vi "Get.vi"(8 "error in (no error)":errorcluster, 9 "Parameter":string, 10 "Request":string, 11 "ByteGSWebAPI-V0 in":refnum<class "ByteGSWebAPI-V0.lvclass">) -> (0 "error out":errorcluster, 3 "ByteGSWebAPI-V0 out":refnum<class "ByteGSWebAPI-V0.lvclass">, 4 "body":string, 6 "headers":string)   [LabVIEW 2019, in "ByteGSWebAPI.lvlib" / "ByteGSWebAPI-V0.lvclass"]
uses:
  ByteGSWebAPI-V0.lvclass
  <vilib>/httpClient/LabVIEWHTTPClient.lvlib
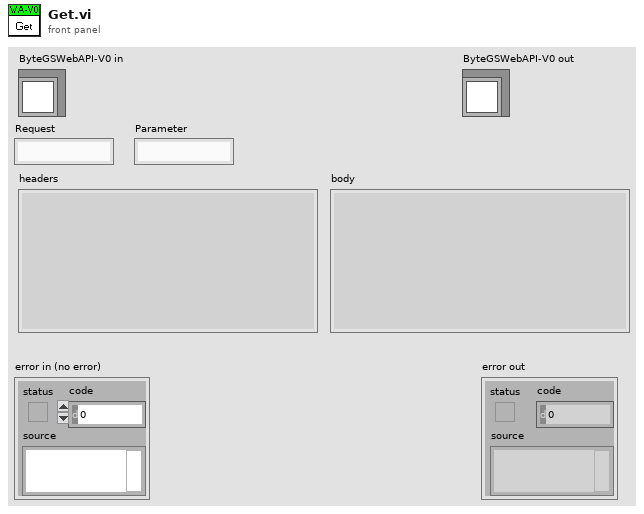
[diagram p1: front panel]
types:
  T1 = typedef "LabVIEWHTTPClient.lvlib/ClientHandle.ctl" = refnum<k1>
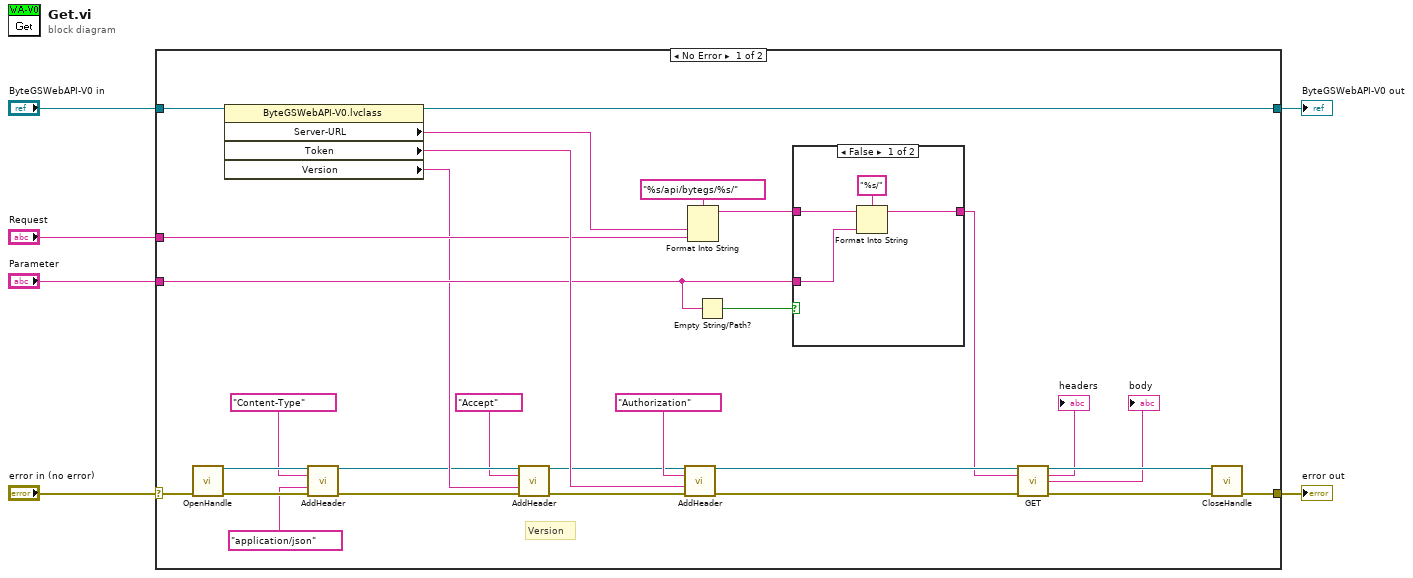
[diagram p0: block diagram]
diagram:
  n1 = case shown="No Error" "error in (no error)" {
    selector: "error in (no error)" -> [w26 w42]
    tunnel: [w25 w42] -> w5
    tunnel: [w24 w41] -> w3
    tunnel: "ByteGSWebAPI-V0 in" -> [w23 w41]
    tunnel: "Request" -> [w17 _]
    tunnel: "Parameter" -> [w13 _]
    frame No Error {
      # "Version"
      n2 = call <vilib>:"OpenHandle.vi"("error in (no error)"=w26) -> ("client handle out"=w31:T1, "error out"=w32:errorcluster)  [unwired: 13 in]
      n3 = property class="ByteGSWebAPI-V0.lvclass"(reference=w23) -> (reference out=w24:refnum<class "ByteGSWebAPI-V0.lvclass">, "Server-URL"=w20:string, "Token"=w22:string, "Version"=w12:string)  [unwired: 1 in, 1 out]
      n4 = call <vilib>:"AddHeader.vi"("client handle"=w31, "header"="Content-Type", "value"="application/json", "error in (no error)"=w32) -> ("client handle out"=w11:T1, "error out"=w10:errorcluster)  [unwired: 10 in]
      n5 = call <vilib>:"AddHeader.vi"("client handle"=w11, "header"="Accept", "value"=w12, "error in (no error)"=w10) -> ("client handle out"=w8:T1, "error out"=w9:errorcluster)  [unwired: 10 in]
      n6 = call <vilib>:"AddHeader.vi"("client handle"=w8, "header"="Authorization", "value"=w22, "error in (no error)"=w9) -> ("client handle out"=w34:T1, "error out"=w33:errorcluster)  [unwired: 10 in]
      n7 = Format Into String(format string="%s/api/bytegs/%s/" ("url"), w20, w17) -> (resulting string=w16:string)  [unwired: 2 in, 1 out]
      n8 = Empty String/Path?(string/path=w13) -> (empty?=w15:bool)
      n9 = case shown="False" w15 {
        tunnel: w16 -> [w38 w40]
        tunnel: [w36 w40] -> w14
        tunnel: w13 -> [w37 _]
        frame False {
          n10 = Format Into String(format string="%s/" ("url"), initial string=w38, w37) -> (resulting string=w36:string)  [unwired: 1 in, 1 out]
        }
        frame True {
        }
      }
      n11 = call <vilib>:"GET.vi"("client handle"=w34, "url"=w14, "error in (no error)"=w33) -> ("client handle out"=w29:T1, "headers"=→"headers":string, "body"=→"body":string, "error out"=w28:errorcluster)  [unwired: 9 in]
      n12 = call <vilib>:"CloseHandle.vi"("client handle"=w29, "error in (no error)"=w28) -> ("error out"=w25:errorcluster)  [unwired: 13 in]
    }
    frame Error {
    }
  }
  "error out" <- w5
  "ByteGSWebAPI-V0 out" <- w3
